vi "SaveGaussGraphs.vi"(10 "XYGraph right":refnum<vi>, 11 "XYGraph left":refnum<vi>) -> ()   [LabVIEW 2013]
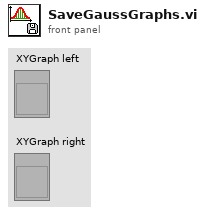
[diagram p1: front panel]
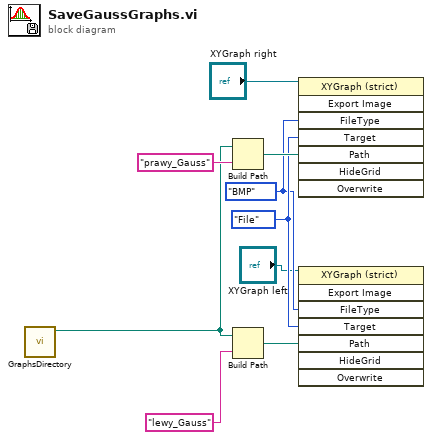
[diagram p0: block diagram]
diagram:
  w5 = enum32{"File", "Clipboard"}."File" ("Target")
  w4 = enum32{"BMP", "EPS", "EMF", "PICT"}."BMP" ("File Type")
  n1 = call "GraphsDirectory.vi"() -> ("dup path"=w1:path)  [unwired: 11 in]
  n2 = Build Path(base path=w1, name or relative path="prawy_Gauss") -> (appended path=w9:path)
  n3 = Build Path(base path=w1, name or relative path="lewy_Gauss") -> (appended path=w7:path)
  n4 = invoke on="Invoke Node" class="XYGraph (strict)" method="Export Image"(reference="XYGraph right", "FileType"=w4, "Target"=w5, "Path"=w9) -> ()  [unwired: 4 in, 8 out]
  n5 = invoke on="Invoke Node" class="XYGraph (strict)" method="Export Image"(reference="XYGraph left", "FileType"=w4, "Target"=w5, "Path"=w7) -> ()  [unwired: 4 in, 8 out]
